vi "Test Assert Less Or Equal.vi"(8 "error in (no error)":errorcluster) -> (0 "error out":errorcluster)   [LabVIEW 2013]
uses:
  classes/Assert/Assert.lvclass
  classes/Test/Test.lvclass
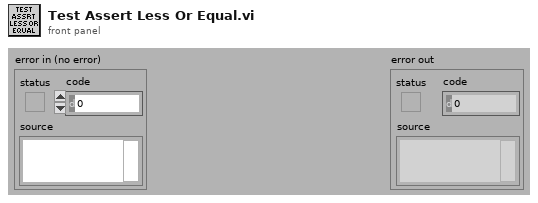
[diagram p1: front panel]
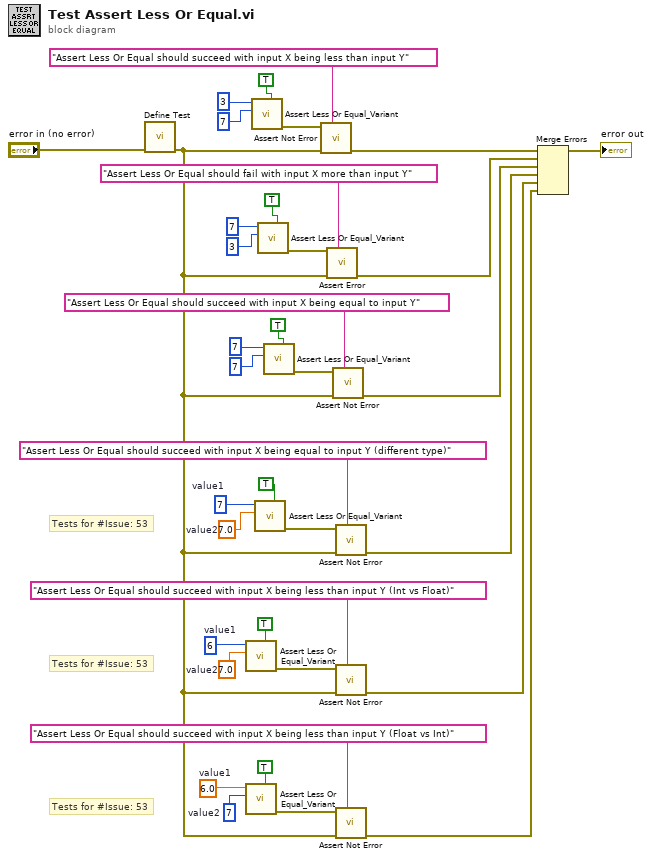
[diagram p0: block diagram]
diagram:
  w6 = 7  # value2
  w5 = 6.0  # value1
  w13 = 7.0  # value2
  w14 = 6  # value1
  w9 = 7.0  # value2
  w10 = 7  # value1
  # "Tests for #Issue: 53"
  # "Tests for #Issue: 53"
  # "Tests for #Issue: 53"
  n1 = call "Define Test.vi"("error in (no error)"="error in (no error)") -> ("error out"=w2:errorcluster)  [unwired: 10 in]
  n2 = call "Assert Less Or Equal_Variant.vi"("Assert Only? (F)"=TRUE, "Y"=w13, "X"=w14) -> ("error out"=w15:errorcluster)  [unwired: 8 in]
  n3 = call "Assert Less Or Equal_Variant.vi"("Assert Only? (F)"=TRUE, "Y"=w6, "X"=w5) -> ("error out"=w4:errorcluster)  [unwired: 8 in]
  n4 = call "Assert Less Or Equal_Variant.vi"("Assert Only? (F)"=TRUE, "Y"=7, "X"=3) -> ("error out"=w39:errorcluster)  [unwired: 8 in]
  n5 = call "Assert Less Or Equal_Variant.vi"("Assert Only? (F)"=TRUE, "Y"=w9, "X"=w10) -> ("error out"=w8:errorcluster)  [unwired: 8 in]
  n6 = call "Assert Less Or Equal_Variant.vi"("Assert Only? (F)"=TRUE, "Y"=3, "X"=7) -> ("error out"=w37:errorcluster)  [unwired: 8 in]
  n7 = call "Assert Less Or Equal_Variant.vi"("Assert Only? (F)"=TRUE, "Y"=7, "X"=7) -> ("error out"=w25:errorcluster)  [unwired: 8 in]
  n8 = call "Assert Not Error.vi"("Label"="Assert Less Or Equal should succeed with input X being less than input Y", "error in (no error)"=w2, "Not Error?"=w39) -> ("error out"=w31:errorcluster)  [unwired: 8 in]
  n9 = call "Assert Error.vi"("Label"="Assert Less Or Equal should fail with input X more than input Y", "error in (no error)"=w2, "Error?"=w37) -> ("error out"=w32:errorcluster)  [unwired: 8 in]
  n10 = call "Assert Not Error.vi"("Label"="Assert Less Or Equal should succeed with input X being equal to input Y", "error in (no error)"=w2, "Not Error?"=w25) -> ("error out"=w20:errorcluster)  [unwired: 8 in]
  n11 = call "Assert Not Error.vi"("Label"="Assert Less Or Equal should succeed with input X being equal to input Y (different type)", "error in (no error)"=w2, "Not Error?"=w8) -> ("error out"=w17:errorcluster)  [unwired: 8 in]
  n12 = call "Assert Not Error.vi"("Label"="Assert Less Or Equal should succeed with input X being less than input Y (Int vs Float)", "error in (no error)"=w2, "Not Error?"=w15) -> ("error out"=w16:errorcluster)  [unwired: 8 in]
  n13 = call "Assert Not Error.vi"("Label"="Assert Less Or Equal should succeed with input X being less than input Y (Float vs Int)", "error in (no error)"=w2, "Not Error?"=w4) -> ("error out"=w1:errorcluster)  [unwired: 8 in]
  n14 = Merge Errors(w31, w32, w20, w17, w16, w1) -> (→"error out":errorcluster)
